vi "Get Aircraft RC Override.vi"(8 "Error In":errorcluster, 11 "Aircraft ID":u8) -> (0 "Error Out":errorcluster, 3 "RC Override Values Out":T1)   [LabVIEW 2014]
uses:
  Controls/RC Override.ctl
  Controls/Aircraft Mode.ctl
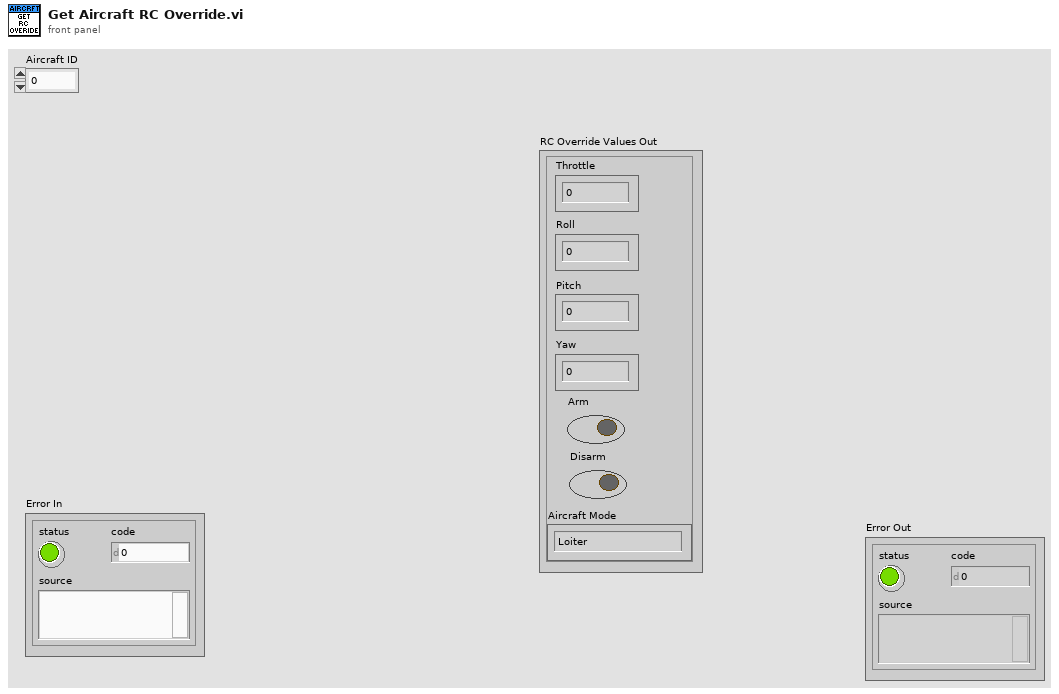
[diagram p1: front panel]
types:
  T1 = typedef "RC Override.ctl" = cluster{"Throttle":u16, "Roll":u16, "Pitch":u16, "Yaw":u16, "Arm":bool, "Disarm":bool, "Aircraft Mode":T2}
  T2 = typedef "Aircraft Mode.ctl" = enum16{"Loiter", "Stabalise", "Failsafe", "Emergency Stop"}
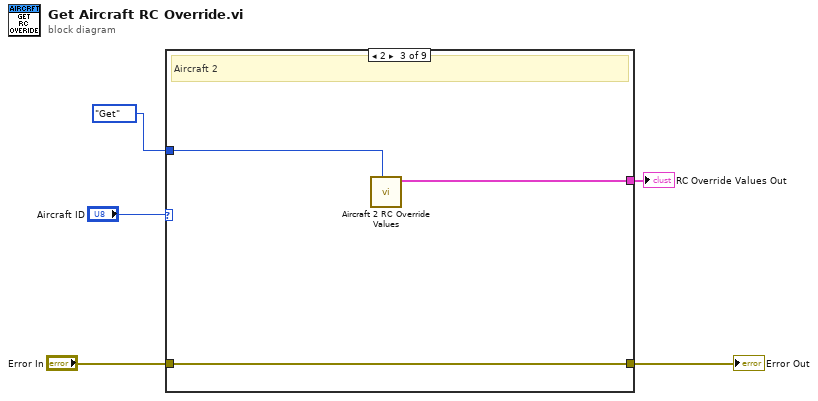
[diagram p0: block diagram]
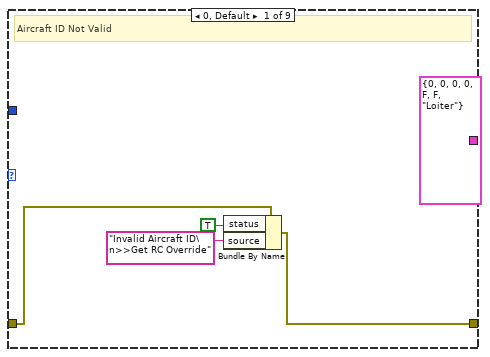
[diagram p2: hidden frame]
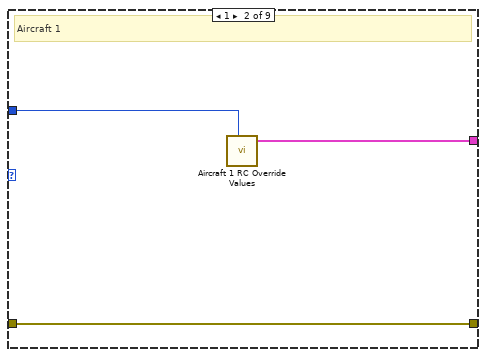
[diagram p3: hidden frame]
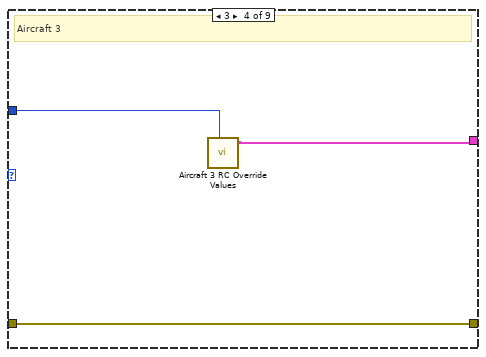
[diagram p4: hidden frame]
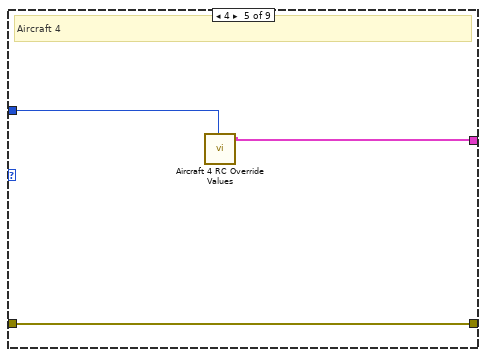
[diagram p5: hidden frame]
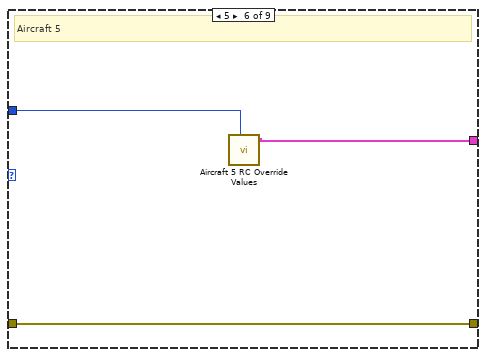
[diagram p6: hidden frame]
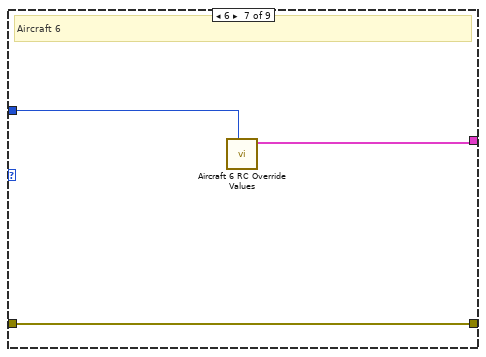
[diagram p7: hidden frame]
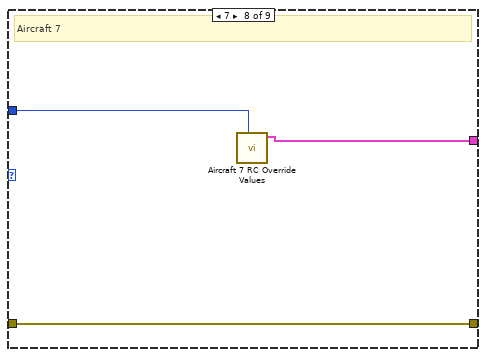
[diagram p8: hidden frame]
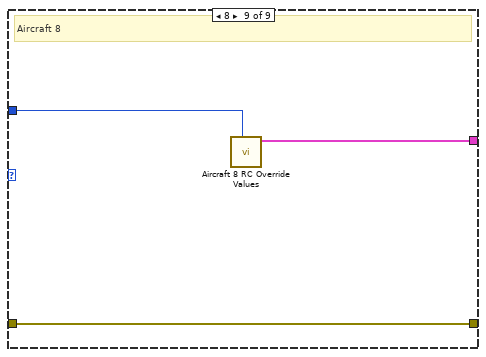
[diagram p9: hidden frame]
diagram:
  n1 = case shown="2" "Aircraft ID" {
    tunnel: [T1 {"Throttle"=0, "Roll"=0, "Pitch"=0, "Yaw"=0, "Arm"=FALSE, "Disarm"=FALSE, "Aircraft Mode"=enum."Loiter"} ("Auto Override Values Out") w12 w15 w18 w21 w24 w27 w30 w33] -> w1
    tunnel: [w9 w13 w16 w19 w22 w25 w28 w31 w34] -> w4
    tunnel: "Error In" -> [w10 w13 w16 w19 w22 w25 w28 w31 w34]
    tunnel: enum16{"Get", "Set"}."Get" ("Method") -> [_ w11 w14 w17 w20 w23 w26 w29 w32]
    frame 0, Default {
      # "Aircraft ID Not Valid"
      n2 = Bundle By Name(cluster=w10, "status"=TRUE, "source"="Invalid Aircraft ID\n>>Get RC Override") -> (w9:errorcluster)
    }
    frame 1 {
      # "Aircraft 1"
      n3 = call "Aircraft 1 RC Override Values.vi"("Method"=w11) -> ("Auto Override Values Out"=w12:T1)  [unwired: 10 in]
    }
    frame 2 {
      # "Aircraft 2"
      n4 = call "Aircraft 2 RC Override Values.vi"("Method"=w14) -> ("Auto Override Values Out"=w15:T1)  [unwired: 10 in]
    }
    frame 3 {
      # "Aircraft 3"
      n5 = call "Aircraft 3 RC Override Values.vi"("Method"=w17) -> ("Auto Override Values Out"=w18:T1)  [unwired: 10 in]
    }
    frame 4 {
      # "Aircraft 4"
      n6 = call "Aircraft 4 RC Override Values.vi"("Method"=w20) -> ("Auto Override Values Out"=w21:T1)  [unwired: 10 in]
    }
    frame 5 {
      # "Aircraft 5"
      n7 = call "Aircraft 5 RC Override Values.vi"("Method"=w23) -> ("Auto Override Values Out"=w24:T1)  [unwired: 10 in]
    }
    frame 6 {
      # "Aircraft 6"
      n8 = call "Aircraft 6 RC Override Values.vi"("Method"=w26) -> ("Auto Override Values Out"=w27:T1)  [unwired: 10 in]
    }
    frame 7 {
      # "Aircraft 7"
      n9 = call "Aircraft 7 RC Override Values.vi"("Method"=w29) -> ("Auto Override Values Out"=w30:T1)  [unwired: 10 in]
    }
    frame 8 {
      # "Aircraft 8"
      n10 = call "Aircraft 8 RC Override Values.vi"("Method"=w32) -> ("Auto Override Values Out"=w33:T1)  [unwired: 10 in]
    }
  }
  "Error Out" <- w4
  "RC Override Values Out" <- w1
